vi "get channel names from typedef.vi"(8 "error in":errorcluster, 10 "channel classification":T1, 11 "fixed channel configuration":refnum<class "control module configuration.lvclass">) -> (0 "error out":errorcluster, 3 "Channel Names":string[](array[string]))   [LabVIEW 2013, in "control module configuration.lvclass"]
uses:
  control module configuration.lvclass
  <vilib>/NI/Tag Bus Module Framework/channel/channel classification.ctl
  <vilib>/Utility/VariantDataType/VariantType.lvlib
  <vilib>/NI/Tag Bus Module Framework/channel/TBM channel.lvclass
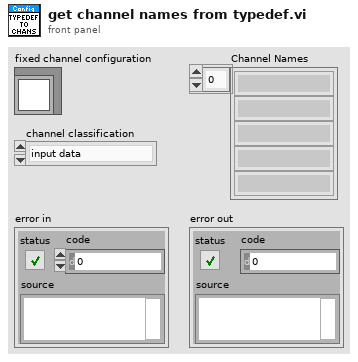
[diagram p1: front panel]
types:
  T1 = typedef "TBM channel.lvclass/channel classification.ctl" = enum16{"input data", "output data", "processing parameter", "processing result"}
  T2 = typedef "control module configuration.lvclass/index type definitions.ctl" = cluster{"input indices":variant, "parameter indices":variant, "result indices":variant, "output indices":variant}
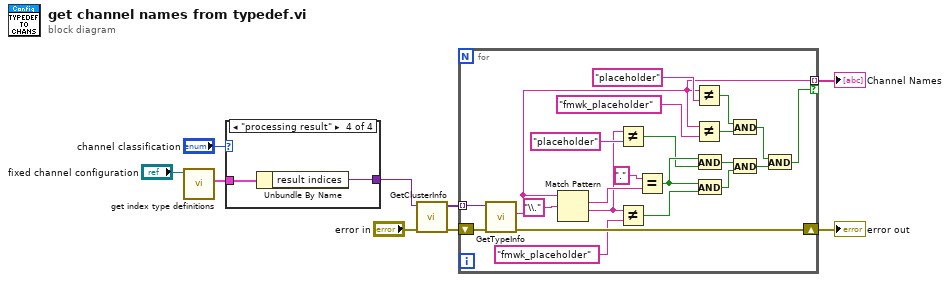
[diagram p0: block diagram]
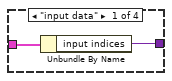
[diagram p2: hidden frame]
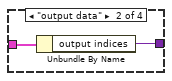
[diagram p3: hidden frame]
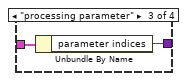
[diagram p4: hidden frame]
diagram:
  n1 = call-dynamic "get index type definitions.vi"("fixed channel configuration in"="fixed channel configuration") -> ("index type defs"=w1:T2)  [unwired: 9 in, 1 out]
  n2 = case shown="\"processing result\"" "channel classification" {
    tunnel: [w10 w12 w14 w16] -> w5
    tunnel: w1 -> [w11 w13 w15 w17]
    frame "input data" {
      n3 = Unbundle By Name(w11) -> ("input indices"=w10:variant)
    }
    frame "output data" {
      n4 = Unbundle By Name(w13) -> ("output indices"=w12:variant)
    }
    frame "processing parameter" {
      n5 = Unbundle By Name(w15) -> ("parameter indices"=w14:variant)
    }
    frame "processing result" {
      n6 = Unbundle By Name(w17) -> ("result indices"=w16:variant)
    }
  }
  n7 = call <vilib>:"GetClusterInfo.vi"("error in (no error)"="error in", "Variant"=w5) -> ("error out"=w7:errorcluster, "Cluster Elements"=w8:variant[])  [unwired: 8 in]
  n8 = for {
    tunnel: w8 -> [w39] mode=indexing
    tunnel: [w31] -> w3 mode=indexing if=w29
    shift-right: [w38] -> w4
    shift-left: w7 -> [w37]
    n9 = call <vilib>:"GetTypeInfo.vi"("error in (no error)"=w37, "Variant"=w39) -> ("error out"=w38:errorcluster, "Name"=w31:string)  [unwired: 5 in, 3 out]
    n10 = Match Pattern(string=w31, regular expression="\\.") -> (match substring=w28:string, after substring=w18:string)  [unwired: 1 in, 2 out]
    n11 = Not Equal?(x=w18, y="placeholder") -> (x != y?=w20:bool)
    n12 = Not Equal?(x=w18, y="fmwk_placeholder") -> (x != y?=w21:bool)
    n13 = Equal?(x=".", y=w28) -> (x = y?=w26:bool)
    n14 = Not Equal?(x=w31, y="placeholder") -> (x != y?=w33:bool)
    n15 = Not Equal?(x=w31, y="fmwk_placeholder") -> (x != y?=w36:bool)
    n16 = And(x=w26, y=w20) -> (x .and. y?=w24:bool)
    n17 = And(x=w26, y=w21) -> (x .and. y?=w25:bool)
    n18 = And(x=w33, y=w36) -> (x .and. y?=w30:bool)
    n19 = And(x=w24, y=w25) -> (x .and. y?=w23:bool)
    n20 = And(x=w30, y=w23) -> (x .and. y?=w29:bool)
  }
  "Channel Names" <- w3
  "error out" <- w4
